vi "rotate_to_face_eye.vi"(2 "Track Eye":T1, 3 "Object To Rotate":refnum<vi>) -> (1 "Rotated Object":refnum<vi>)   [LabVIEW 2020, in "3DPC_SurfacePlot.xctl"]
uses:
  <vilib>/Native 3D Graph/xcontrol/3DPC_SurfacePlot.xctl
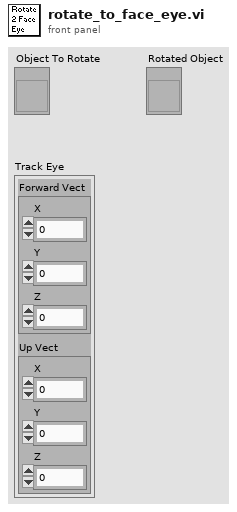
[diagram p1: front panel]
types:
  T1 = cluster{"Forward Vect":cluster{"X":dbl, "Y":dbl, "Z":dbl}, "Up Vect":cluster{"X":dbl, "Y":dbl, "Z":dbl}}
  T2 = cluster{"A x Vector[0]":dbl, "A x Vector[1]":dbl, "A x Vector[2]":dbl}
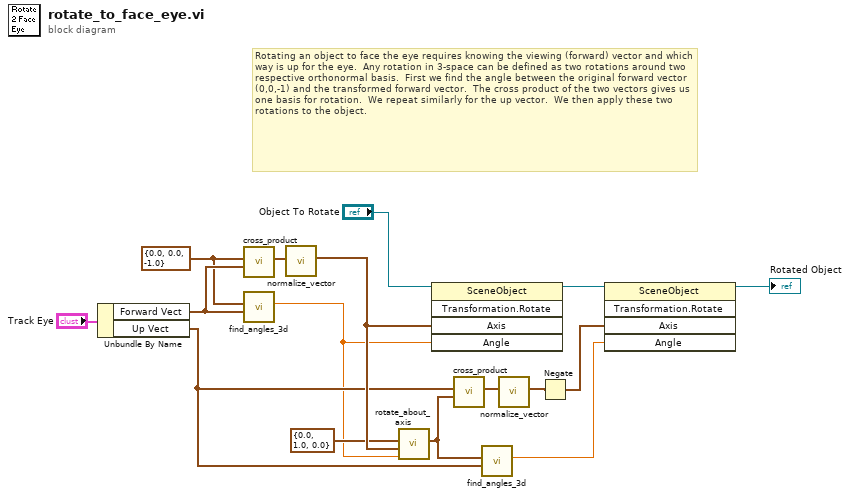
[diagram p0: block diagram]
diagram:
  w11 = cluster{"X":dbl, "Y":dbl, "Z":dbl} {"X"=0.0, "Y"=0.0, "Z"=-1.0} ("Vect 1")
  # "Rotating an object to face the eye requires knowing the viewing (forward) vector and which way is up for the eye.  Any rotation in 3-space can be defined as two rotations around two respective orthonormal basis.  First we find the angle between the original forward vector (0,0,-1) and the transformed forward vector.  The cross product of the two vectors gives us one basis for rotation.  We repeat similarly for the up vector.  We then apply these two rotations to the object."
  n1 = Unbundle By Name("Track Eye") -> ("Forward Vect"=w14:cluster{"X":dbl, "Y":dbl, "Z":dbl}, "Up Vect"=w7:cluster{"X":dbl, "Y":dbl, "Z":dbl})
  n2 = call <vilib>:"cross_product.vi"("Vect 2"=w14, "Vect 1"=w11) -> ("Vect Out"=w2:cluster{"X":sgl, "Y":sgl, "Z":sgl})  [unwired: 9 out]
  n3 = call <vilib>:"find_angles_3d.vi"("Vect 2"=w14, "Vect 1"=w11) -> ("angle"=w4:dbl)  [unwired: 9 out]
  n4 = call <vilib>:"normalize_vector.vi"("Vector"=w2) -> ("Normalized Vector"=w12:cluster{"X":sgl, "Y":sgl, "Z":sgl})  [unwired: 10 out]
  n5 = call <vilib>:"rotate_about_axis.vi"("Angle"=w4, "Axis"=w12, "Vector"=cluster{"X":dbl, "Y":dbl, "Z":dbl} {"X"=0.0, "Y"=1.0, "Z"=0.0} ("Vect 1")) -> ("Rotated Vector"=w8:T2)  [unwired: 8 out]
  n6 = invoke class="SceneObject" method="Transformation.Rotate"(reference="Object To Rotate", "Axis"=w12, "Angle"=w4) -> (reference out=w9:refnum<vi>)  [unwired: 2 in, 4 out]
  n7 = call <vilib>:"cross_product.vi"("Vect 2"=w8, "Vect 1"=w7) -> ("Vect Out"=w5:cluster{"X":sgl, "Y":sgl, "Z":sgl})  [unwired: 9 out]
  n8 = call <vilib>:"find_angles_3d.vi"("Vect 2"=w7, "Vect 1"=w8) -> ("angle"=w3:dbl)  [unwired: 9 out]
  n9 = call <vilib>:"normalize_vector.vi"("Vector"=w5) -> ("Normalized Vector"=w15:cluster{"X":sgl, "Y":sgl, "Z":sgl})  [unwired: 10 out]
  n10 = Negate(x=w15) -> (-x=w13:cluster{"X":sgl, "Y":sgl, "Z":sgl})
  n11 = invoke class="SceneObject" method="Transformation.Rotate"(reference=w9, "Axis"=w13, "Angle"=w3) -> (reference out=→"Rotated Object":refnum<vi>)  [unwired: 2 in, 4 out]
